vi "Get Properties from Selected Item.vi"(7 "Action":T3, 8 "Error In":errorcluster, 11 "Affected Items":T4) -> (0 "Error Out":errorcluster, 1 "Property Array Out":T1(array[cluster]), 2 "Use Dialog?":bool, 3 "Properties for Tree Out":T2(array[cluster]))   [LabVIEW 2023]
doc: "Return properties from any terminal, wire or property node. Returns all properties for insert and drop actions, and displayed properties for remove and rearrange actions.\n\nThis is amazing,. because it relies on creating a temporary property node to get all available properties. I think we could also get these from our helper file more quickly. (The current method isn't terribly slow, though.)"
uses:
  top/BundleMagic.ctl
  controls/action enum.ctl
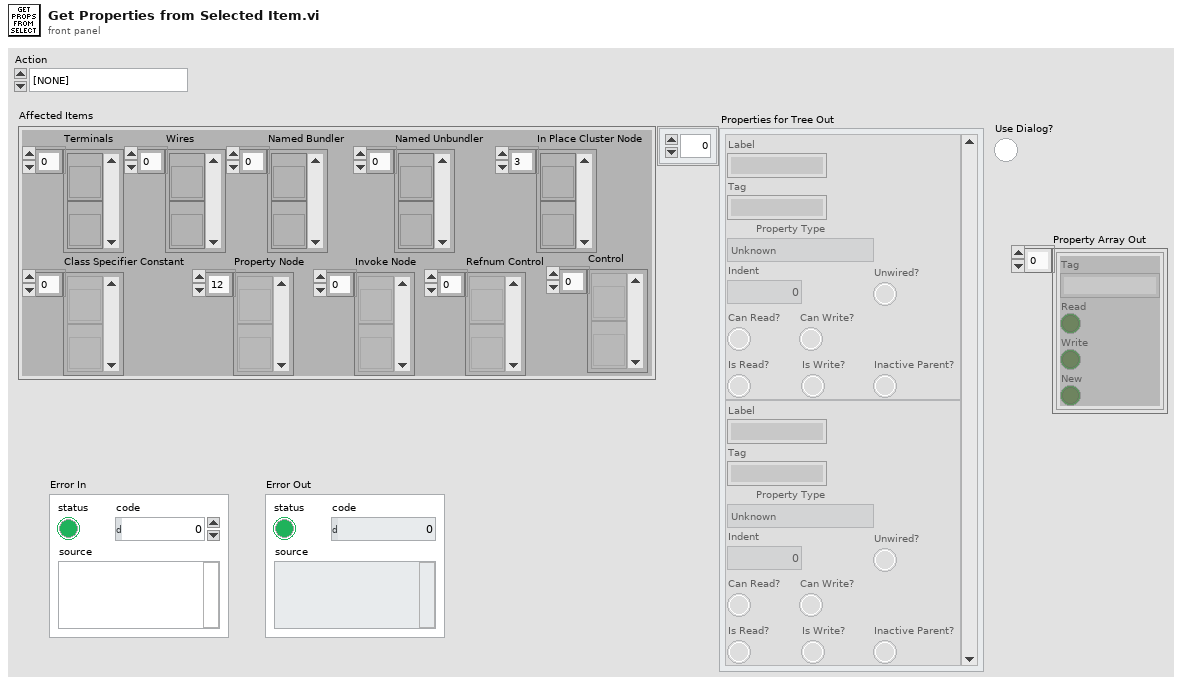
[diagram p1: front panel]
types:
  T1 = cluster{"Tag":string, "Read":bool, "Write":bool, "New":bool}[]
  T2 = cluster{"Label":string, "Tag":string, "Property Type":enum16{"Unknown", "Base", "Scripting", "Private", "Deprecated", "None", "Divider"}, "Indent":u16, "Can Read?":bool, "Can Write?":bool, "Is Read?":bool, "Is Write?":bool, "Inactive Parent?":bool, "Unwired?":bool}[]
  T3 = typedef "action enum.ctl" = enum16{"[NONE]", "Wire Bundle", "Wire Unbundle", "Terminal Unbundle", "Terminal Bundle", "Bundler Move Up", "Bundler Move Down", "Bundler Insert", "Bundler Remove", "Bundler Remove Unwired", "Bundler Rearrange", "In Place Insert", "In Place Remove", "In Place Remove Unwired", "In Place Rearrange", "Wire Properties", "Wire Method", "Terminal Properties", "Terminal Method", "Property Move Up", "Property Move Down", "Properties Insert", "Properties Remove", "Properties Remove Unwired", "Properties Rearrange", "Method Change", "Class for Constant", "Class For Control", "Class For Node", "Class Name to Clipboard"}
  T4 = typedef "BundleMagic.ctl" = cluster{"Terminals":refnum<vi>[], "Wires":refnum<vi>[], "Named Bundler":refnum<vi>[], "Named Unbundler":refnum<vi>[], "In Place Cluster Node":refnum<vi>[], "Class Specifier Constant":refnum<vi>[], "Property Node":refnum<vi>[], "Invoke Node":refnum<vi>[], "Refnum Control":refnum<vi>[], "Control":refnum<vi>[]}
  T5 = cluster{"Property/Method Info":cluster{"Unique ID string":string, "Data name":string, "Short name (localized)":string, "Long name (localized)":string}, "Is Write":bool, "Unwired":bool, "Deprecated":bool}
  T6 = cluster{"Property/Method Info":cluster{"Unique ID string":string, "Data name":string, "Short name (localized)":string, "Long name (localized)":string}, "Is Write":bool, "Unwired":bool, "Deprecated":bool}[]
  T7 = cluster{"Unique ID string":string, "Data name":string, "Short name (localized)":string, "Long name (localized)":string}[]
  T8 = typedef "ASPM_ArrayOfUniqueIDStringDatanameShortnameLongname.ctl" = T9[]
  T9 = typedef "ASPM_UniqueIDStringDatanameShortnameLongname.ctl" = cluster{"Unique ID string":string, "Data name":string, "Short name (localized)":string, "Long name (localized)":string}
  T10 = cluster{"Tag":string, "Read":bool, "Write":bool, "New":bool}
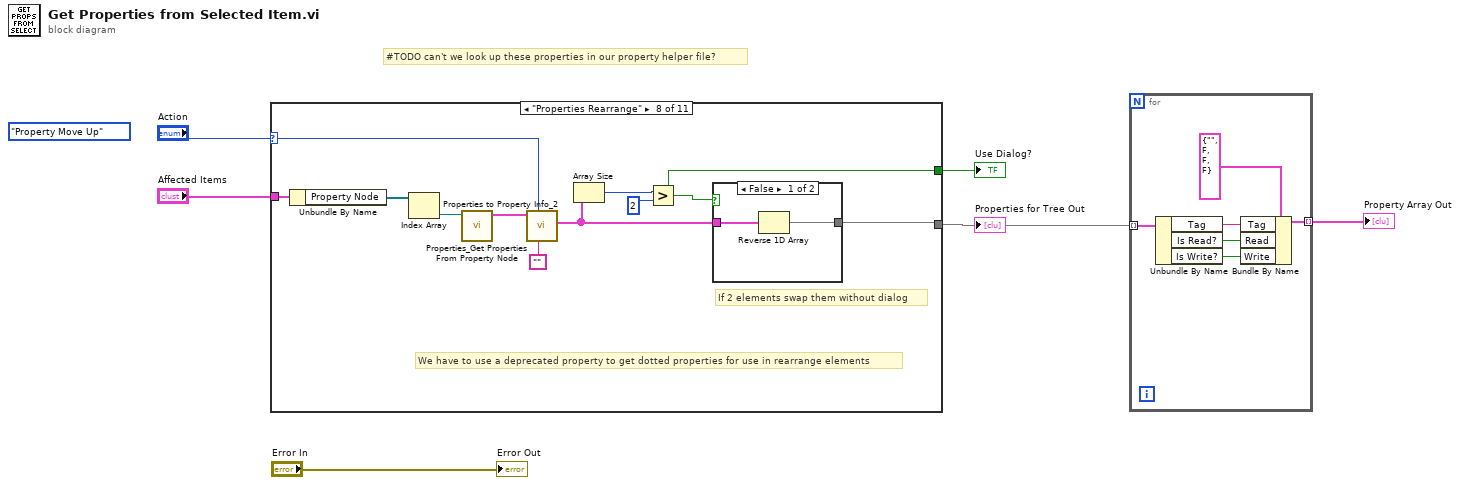
[diagram p0: block diagram]
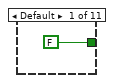
[diagram p2: hidden frame]
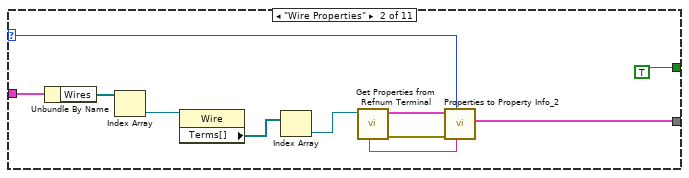
[diagram p3: hidden frame]
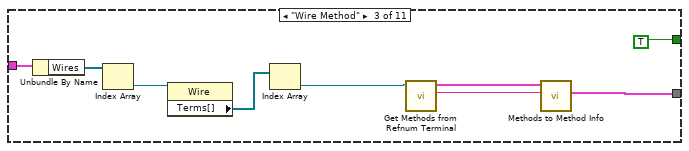
[diagram p4: hidden frame]
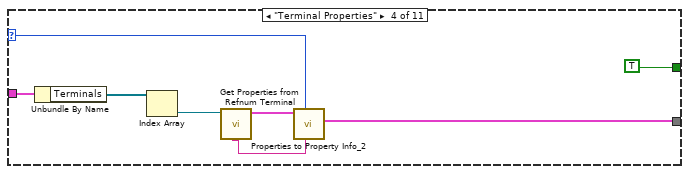
[diagram p5: hidden frame]
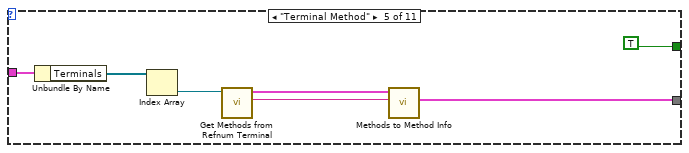
[diagram p6: hidden frame]
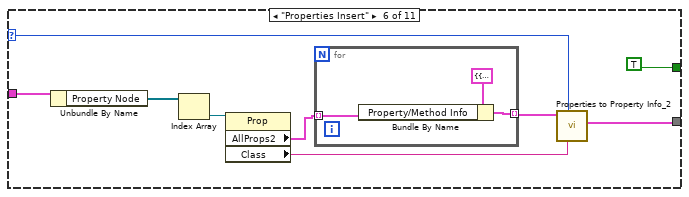
[diagram p7: hidden frame]
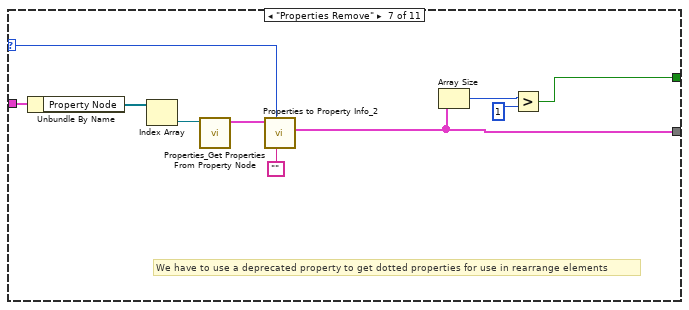
[diagram p8: hidden frame]
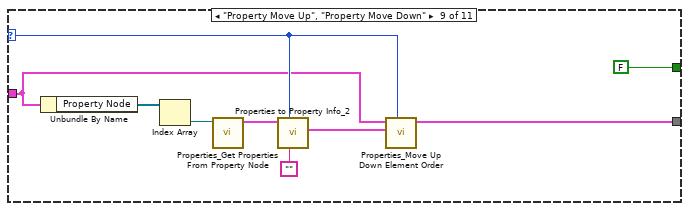
[diagram p10: hidden frame]
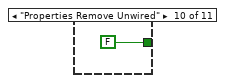
[diagram p11: hidden frame]
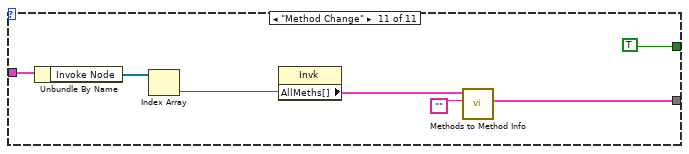
[diagram p12: hidden frame]
diagram:
  (unwired) action_enum."Property Move Up" ("Action")
  # "#TODO can't we look up these properties in our property helper file?"
  n1 = case shown="\"Properties Rearrange\"" "Action" {
    selector: "Action" -> [_ w12 _ w31 _ w47 w62 w73 w80 _ _]
    tunnel: "Affected Items" -> [_ w18 w24 w35 w42 w49 w64 w75 w79 _ w93]
    tunnel: [_ w11 w21 w30 w38 w48 w58 w65 w81 _ w91] -> w2
    tunnel: [FALSE TRUE TRUE TRUE TRUE TRUE w55 w67 FALSE FALSE TRUE] -> w3
    frame Default {
    }
    frame "Wire Properties" {
      n2 = Unbundle By Name(w18) -> ("Wires"=w17:refnum<vi>[])
      n3 = Index Array(array=w17) -> (element=w16:refnum<vi>)  [unwired: 1 in]
      n4 = property class="Wire"(reference=w16) -> ("Terms[]"=w15:refnum<vi>[])  [unwired: 1 in, 2 out]
      n5 = Index Array(array=w15) -> (element=w14:refnum<vi>)  [unwired: 1 in]
      n6 = call "Get Properties from Refnum Terminal.vi"("Refnum Terminal"=w14) -> ("error out"=w10:errorcluster, "All Properties for Refnum Terminal"=w13:T6, "Class"=w9:string)  [unwired: 7 in, 1 out]
      n7 = call "Properties to Property Info_2.vi"("Class"=w9, "Action"=w12, "Error In"=w10, "All Properties for Refnum Terminal"=w13) -> ("Properties for Tree Out"=w11:T2)  [unwired: 5 in, 2 out]
    }
    frame "Wire Method" {
      n8 = Unbundle By Name(w24) -> ("Wires"=w27:refnum<vi>[])
      n9 = Index Array(array=w27) -> (element=w26:refnum<vi>)  [unwired: 1 in]
      n10 = property class="Wire"(reference=w26) -> ("Terms[]"=w25:refnum<vi>[])  [unwired: 1 in, 2 out]
      n11 = Index Array(array=w25) -> (element=w23:refnum<vi>)  [unwired: 1 in]
      n12 = call "Get Methods from Refnum Terminal.vi"("Refnum Terminal"=w23) -> ("Class"=w20:string, "All Methods for Refnum Terminal"=w22:T7)  [unwired: 8 in, 1 out]
      n13 = call "Methods to Method Info.vi"("Class"=w20, "Methods from Node"=w22) -> ("Methods for Tree"=w21:T2)  [unwired: 8 in, 1 out]
    }
    frame "Terminal Properties" {
      n14 = Unbundle By Name(w35) -> ("Terminals"=w34:refnum<vi>[])
      n15 = Index Array(array=w34) -> (element=w33:refnum<vi>)  [unwired: 1 in]
      n16 = call "Get Properties from Refnum Terminal.vi"("Refnum Terminal"=w33) -> ("All Properties for Refnum Terminal"=w32:T6, "Class"=w29:string)  [unwired: 7 in, 2 out]
      n17 = call "Properties to Property Info_2.vi"("Class"=w29, "Action"=w31, "All Properties for Refnum Terminal"=w32) -> ("Properties for Tree Out"=w30:T2)  [unwired: 6 in, 2 out]
    }
    frame "Terminal Method" {
      n18 = Unbundle By Name(w42) -> ("Terminals"=w41:refnum<vi>[])
      n19 = Index Array(array=w41) -> (element=w40:refnum<vi>)  [unwired: 1 in]
      n20 = call "Get Methods from Refnum Terminal.vi"("Refnum Terminal"=w40) -> ("Class"=w37:string, "All Methods for Refnum Terminal"=w39:T7)  [unwired: 8 in, 1 out]
      n21 = call "Methods to Method Info.vi"("Class"=w37, "Methods from Node"=w39) -> ("Methods for Tree"=w38:T2)  [unwired: 8 in, 1 out]
    }
    frame "Properties Insert" {
      n22 = Unbundle By Name(w49) -> ("Property Node"=w51:refnum<vi>[])
      n23 = Index Array(array=w51) -> (element=w50:refnum<vi>)  [unwired: 1 in]
      n24 = property class="Prop"(reference=w50) -> ("AllProps2"=w45:T8, "Class"=w46:string)  [unwired: 1 in, 2 out]
      n25 = for {
        tunnel: w45 -> [w53] mode=indexing
        tunnel: [w52] -> w44 mode=indexing
        n26 = Bundle By Name(cluster=T5 {"Property/Method Info"={"Unique ID string"="", "Data name"="", "Short name (localized)"="", "Long name (localized)"=""}, "Is Write"=FALSE, "Unwired"=FALSE, "Deprecated"=FALSE} ("Cluster"), "Property/Method Info"=w53) -> (w52:T5)
      }
      n27 = call "Properties to Property Info_2.vi"("Class"=w46, "Action"=w47, "All Properties for Refnum Terminal"=w44) -> ("Properties for Tree Out"=w48:T2)  [unwired: 6 in, 2 out]
    }
    frame "Properties Remove" {
      # "We have to use a deprecated property to get dotted properties for use in rearrange elements"
      n28 = Unbundle By Name(w64) -> ("Property Node"=w63:refnum<vi>[])
      n29 = Index Array(array=w63) -> (element=w60:refnum<vi>)  [unwired: 1 in]
      n30 = call "Properties_Get Properties From Property Node.vi"("Property in"=w60) -> ("All Properties for Refnum Terminal"=w59:T6)  [unwired: 10 in]
      n31 = call "Properties to Property Info_2.vi"("Class"="", "Action"=w62, "All Properties for Refnum Terminal"=w59) -> ("Properties for Tree Out"=w58:T2)  [unwired: 6 in, 2 out]
      n32 = Array Size(array=w58) -> (size(s)=w57:i32)
      n33 = Greater?(x=w57, y=1) -> (0:w55:bool)
    }
    frame "Properties Rearrange" {
      # "If 2 elements swap them without dialog"
      # "We have to use a deprecated property to get dotted properties for use in rearrange elements"
      n34 = Unbundle By Name(w75) -> ("Property Node"=w74:refnum<vi>[])
      n35 = Index Array(array=w74) -> (element=w71:refnum<vi>)  [unwired: 1 in]
      n36 = call "Properties_Get Properties From Property Node.vi"("Property in"=w71) -> ("All Properties for Refnum Terminal"=w70:T6)  [unwired: 10 in]
      n37 = call "Properties to Property Info_2.vi"("Class"="", "Action"=w73, "All Properties for Refnum Terminal"=w70) -> ("Properties for Tree Out"=w66:T2)  [unwired: 6 in, 2 out]
      n38 = Array Size(array=w66) -> (size(s)=w69:i32)
      n39 = Greater?(x=w69, y=2) -> (0:w67:bool)
      n40 = case shown="False" w67 {
        tunnel: [w76 w78] -> w65
        tunnel: w66 -> [w77 w78]
        frame False {
          n41 = Reverse 1D Array(array=w77) -> (reversed array=w76:T2)
        }
        frame True {
        }
      }
    }
    frame "Property Move Up", "Property Move Down" {
      n42 = Unbundle By Name(w79) -> ("Property Node"=w86:refnum<vi>[])
      n43 = Index Array(array=w86) -> (element=w84:refnum<vi>)  [unwired: 1 in]
      n44 = call "Properties_Get Properties From Property Node.vi"("Property in"=w84) -> ("All Properties for Refnum Terminal"=w83:T6)  [unwired: 10 in]
      n45 = call "Properties to Property Info_2.vi"("Class"="", "Action"=w80, "All Properties for Refnum Terminal"=w83) -> ("Properties for Tree Out"=w82:T2)  [unwired: 6 in, 2 out]
      n46 = call "Properties_Move Up Down Element Order.vi"("Action"=w80, "Properties for Tree Out"=w82, "Affected Items"=w79) -> ("Properties for Tree Out"=w81:T2)  [unwired: 8 in]
    }
    frame "Properties Remove Unwired" {
    }
    frame "Method Change" {
      n47 = Unbundle By Name(w93) -> ("Invoke Node"=w95:refnum<vi>[])
      n48 = Index Array(array=w95) -> (element=w94:refnum<vi>)  [unwired: 1 in]
      n49 = property class="Invk"(reference=w94) -> ("AllMeths[]"=w92:T8)  [unwired: 1 in, 2 out]
      n50 = call "Methods to Method Info.vi"("Class"="", "Methods from Node"=w92) -> ("Methods for Tree"=w91:T2)  [unwired: 8 in, 1 out]
    }
  }
  "Properties for Tree Out" <- w2
  "Use Dialog?" <- w3
  n51 = for {
    tunnel: w2 -> [w101] mode=indexing
    tunnel: [w96] -> w1 mode=indexing
    n52 = Unbundle By Name(w101) -> ("Tag"=w99:string, "Is Read?"=w98:bool, "Is Write?"=w97:bool)
    n53 = Bundle By Name(cluster=T10 {"Tag"="", "Read"=FALSE, "Write"=FALSE, "New"=FALSE} ("Property Tree Element Value"), "Tag"=w99, "Read"=w98, "Write"=w97) -> (w96:T10)
  }
  "Property Array Out" <- w1
  "Error Out" <- "Error In"
